vi "SVGlobal_StatusStop.vi"() -> ()   [LabVIEW 2020, in "Shared Variable Interface.lvlib"]
uses:
  Shared Variable Interface.lvlib
panel:
  in  "StatusStop":bool
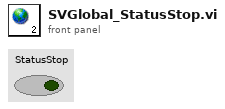
[diagram p1: front panel]
diagram:
